vi "Control Panel.vi"() -> ()   [LabVIEW 2023]
panel:
  in  "Remove Positions":bool
  in  "System Summary":bool
  in  "Add Positions":bool
  in  "Exit":bool
  # "Main Controls"
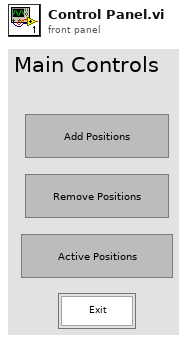
[diagram p1: front panel]
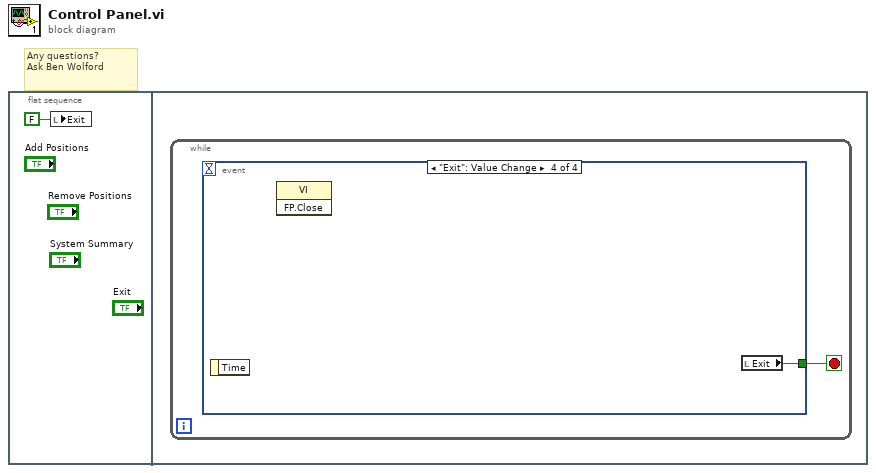
[diagram p0: block diagram]
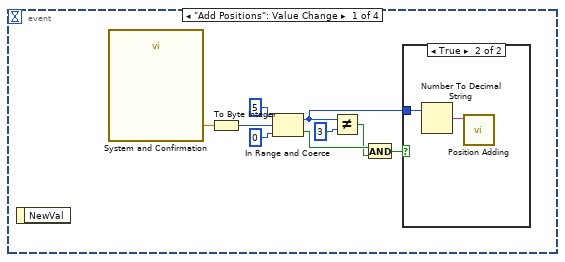
[diagram p2: hidden frame]
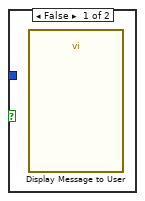
[diagram p3: hidden frame]
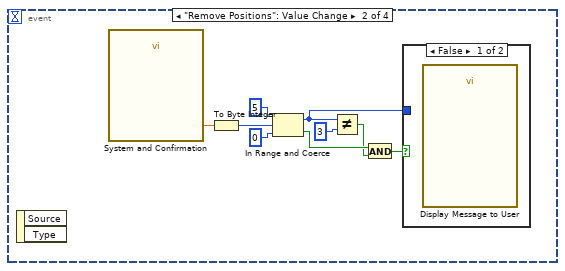
[diagram p4: hidden frame]
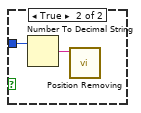
[diagram p5: hidden frame]
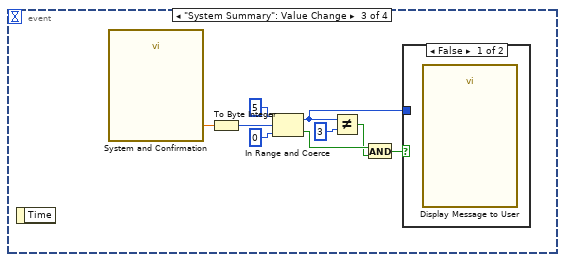
[diagram p6: hidden frame]
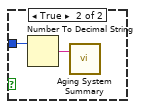
[diagram p7: hidden frame]
diagram:
  # "Any questions?\nAsk Ben Wolford"
  n1 = flat-sequence {
    frame #0 {
      n2 = local write "Exit"(FALSE ("Exit")) -> ()
    }
    frame #1 {
      n3 = while {
        stop <- w2 stop-if-true
        n4 = event shown="[3] \"Exit\": Value Change" {
          selector: _ -> [_ _ _ _]
          dyn-events: _ -> [_ _ _ _]
          timeout: _ -> [_ _ _ _]
          tunnel: [_ _ _ w36] -> w2
          event "Add Positions": Value Change {
            n5 = event-data() -> ()  [unwired: 1 in, 1 out]
            n6 = call "System and Confirmation"() -> ("System"=w10:dbl)  [unwired: 17 in, 2 out]
            n7 = To Byte Integer(number=w10) -> (8bit integer=w11:i8)
            n8 = In Range and Coerce(upper limit=i8 5, x=w11, lower limit=i8 0) -> (coerced(x)=w5:i8, In Range?=w7:bool)
            n9 = Not Equal?(x=w5, y=i8 3) -> (x != y?=w6:bool)
            n10 = And(x=w7, y=w6) -> (x .and. y?=w3:bool)
            n11 = case shown="True" w3 {
              tunnel: w5 -> [_ w13]
              frame False {
                n12 = call "Display Message to User"() -> ()  [unwired: 10 in, 2 out]
              }
              frame True {
                n13 = Number To Decimal String(number=w13) -> (decimal integer string=w12:string)  [unwired: 1 in]
                n14 = call "Position Adding.vi"("System"=w12) -> ()  [unwired: 11 in]
              }
            }
          }
          event "Remove Positions": Value Change {
            n15 = event-data() -> ()  [unwired: 1 in, 2 out]
            n16 = call "System and Confirmation"() -> ("System"=w21:dbl)  [unwired: 17 in, 2 out]
            n17 = To Byte Integer(number=w21) -> (8bit integer=w22:i8)
            n18 = In Range and Coerce(upper limit=i8 5, x=w22, lower limit=i8 0) -> (coerced(x)=w15:i8, In Range?=w17:bool)
            n19 = Not Equal?(x=w15, y=i8 3) -> (x != y?=w16:bool)
            n20 = And(x=w17, y=w16) -> (x .and. y?=w14:bool)
            n21 = case shown="False" w14 {
              tunnel: w15 -> [_ w24]
              frame False {
                n22 = call "Display Message to User"() -> ()  [unwired: 10 in, 2 out]
              }
              frame True {
                n23 = Number To Decimal String(number=w24) -> (decimal integer string=w23:string)  [unwired: 1 in]
                n24 = call "Position Removing.vi"("System"=w23) -> ()  [unwired: 11 in]
              }
            }
          }
          event "System Summary": Value Change {
            n25 = event-data() -> ()  [unwired: 1 in, 1 out]
            n26 = call "System and Confirmation"() -> ("System"=w32:dbl)  [unwired: 17 in, 2 out]
            n27 = To Byte Integer(number=w32) -> (8bit integer=w33:i8)
            n28 = In Range and Coerce(upper limit=i8 5, x=w33, lower limit=i8 0) -> (coerced(x)=w25:i8, In Range?=w27:bool)
            n29 = Not Equal?(x=w25, y=i8 3) -> (x != y?=w26:bool)
            n30 = And(x=w27, y=w26) -> (x .and. y?=w28:bool)
            n31 = case shown="False" w28 {
              tunnel: w25 -> [_ w34]
              frame False {
                n32 = call "Display Message to User"() -> ()  [unwired: 10 in, 2 out]
              }
              frame True {
                n33 = Number To Decimal String(number=w34) -> (decimal integer string=w35:string)  [unwired: 1 in]
                n34 = call "Aging System Summary.vi"("System"=w35) -> ()  [unwired: 2 in]
              }
            }
          }
          event "Exit": Value Change {
            n35 = event-data() -> ()  [unwired: 1 in, 1 out]
            n36 = invoke class="VI" method="FP.Close"() -> ()  [unwired: 3 in, 3 out]
            n37 = local read "Exit"() -> (w36:bool)
          }
        }
      }
    }
  }
